vi "Read.Initialize.vi"(8 "error in":errorcluster, 10 "PluginAPIs":T1=refnum, 11 "Settings":cluster{"Refs":T2[], "Values":dbl[]} {"Refs"."Data Reference" format="%.0x"}) -> (0 "error out":errorcluster, 3 "Read out":refnum<class "Read.lvclass">)   [LabVIEW 2023, in "Plugin Data Access Engine.lvlib" / "Read.lvclass"]
uses:
  Read.lvclass
  Read.lvclass/Read.ctl
  <vilib>/NI VeriStand/Custom Device API/Data Reference.ctl
  <vilib>/NI VeriStand/Custom Device API/Block Data Reference.ctl
  <userlib>/PluginCore_v1.lvlibp/iPluginAPIs/iPluginAPIs.lvclass
  _PluginCore/Types/Plugin API.ctl
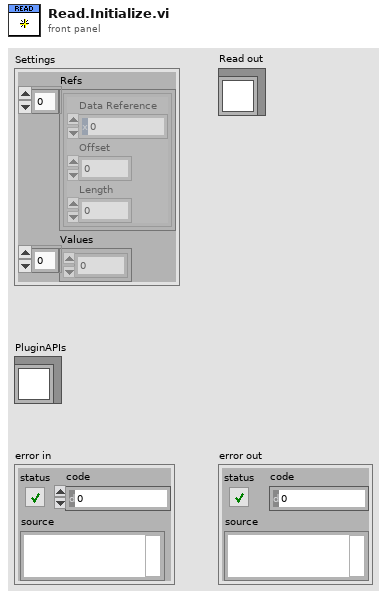
[diagram p1: front panel]
types:
  T1 = typedef "Plugin API.ctl" = refnum<class "iPluginAPIs.lvclass">
  T2 = typedef "Custom Device API.lvlib/Block Data Reference.ctl" = cluster{"Data Reference":T3, "Offset":u64, "Length":u64}
  T3 = typedef "Custom Device API.lvlib/Data Reference.ctl" = i32
  T4 = cluster{"read mode":enum16{"polling", "blocking"}, "write mode":enum16{"polling", "blocking"}}
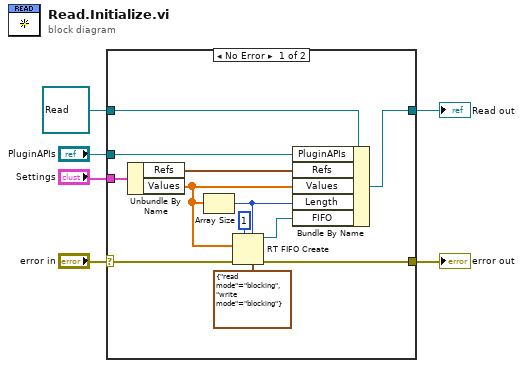
[diagram p0: block diagram]
diagram:
  n1 = case shown="No Error" "error in" {
    selector: "error in" -> [w12 w20]
    tunnel: [w16 w20] -> w6
    tunnel: "Settings" -> [w14 _]
    tunnel: [w13 w19] -> w3
    tunnel: refnum<class "Read.lvclass"> refnum ("Read out") -> [w9 w19]
    tunnel: "PluginAPIs" -> [w7 _]
    frame No Error {
      n2 = Unbundle By Name(w14) -> ("Refs"=w11:T2[], "Values"=w10:dbl[])
      n3 = Array Size(array=w10) -> (size(s)=w8:i32)
      n4 = RT FIFO Create(1:w10, 3:w12, 4:u32 1 ("size (10)"), 6:w8, 7:T4 {"read mode"=enum."blocking", "write mode"=enum."blocking"} ("r/w modes (polling,polling)")) -> (8:w18:refnum<k33>, 11:w16:errorcluster)  [unwired: 3 in, 1 out]
      n5 = Bundle By Name(cluster=w9, "PluginAPIs"=w7, "Refs"=w11, "Values"=w10, "Length"=w8, "FIFO"=w18) -> (w13:refnum<class "Read.lvclass">)
    }
    frame Error {
    }
  }
  "error out" <- w6
  "Read out" <- w3
